vi "Colorbar2004.vi"   [LabVIEW 2013]
uses:
  <vilib>/Heliosphere Research LLC/Advanced Plotting Toolkit/Advanced Plotting Toolkit.lvlib
types:
  T1 = typedef "Advanced Plotting Toolkit.lvlib/PlotID.ctl" = i32
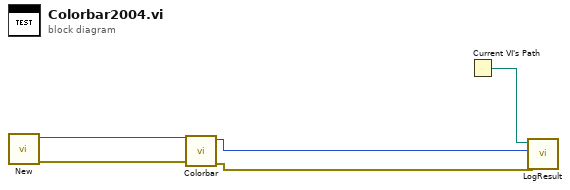
[diagram p0: block diagram]
diagram:
  n1 = call <vilib>:"New.vi"() -> ("error out"=w1:errorcluster, "Plot ID"=w2:T1)  [unwired: 10 in]
  n2 = call <vilib>:"Colorbar.vi"("error in (no error)"=w1, "Plot ID"=w2) -> ("error out"=w4:errorcluster, "Plot ID Out"=w3:T1)  [unwired: 8 in]
  n3 = Current VI's Path() -> (path=w5:path)
  n4 = call "LogResult.vi"("Test Result"=w4, "Test Artifact"=w3, "VI Path"=w5) -> ()  [unwired: 9 in]
